vi "table_control.vi"() -> ()   [LabVIEW 2018]
uses:
  <vilib>/Utility/miscctls.llb/LVRowAndColumnUnsignedTypeDef.ctl
panel:
  in  "Stop":bool
  out "Loop Index":i32
  in  "Table Control":string[][](table)
  # "Adapted from\nhttps://www.youtube.com/watch?v=RbDLJ1aaG3E"
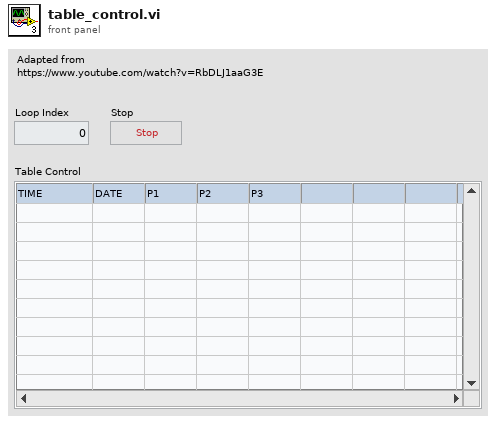
[diagram p1: front panel]
types:
  T1 = typedef "LVRowAndColumnUnsignedTypeDef.ctl" = cluster{"Row":u32, "Column":u32}
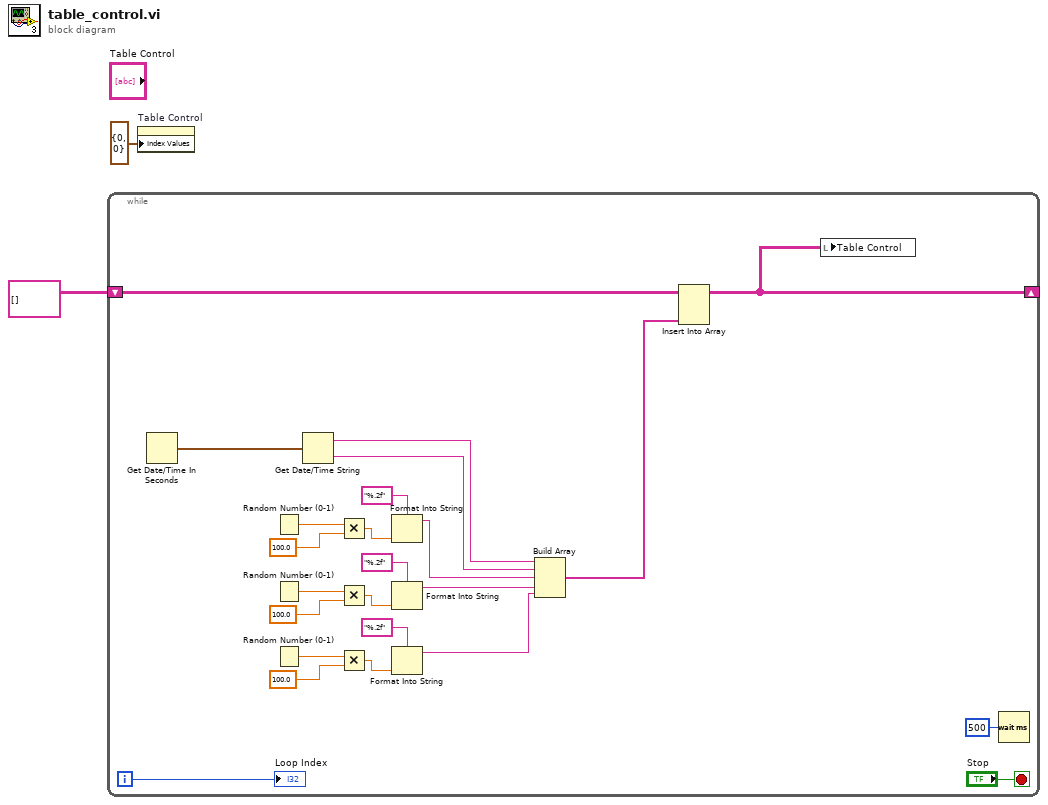
[diagram p0: block diagram]
diagram:
  n1 = while {
    shift-right: [w24] -> _
    shift-left: string[][] [] -> [w25]
    i -> [w26]
    stop <- "Stop" stop-if-true
    n2 = Get Date/Time In Seconds() -> (seconds since 1Jan1904=w6:timestamp)
    n3 = Random Number (0-1)() -> (number: 0 to 1=w23:dbl)
    n4 = Random Number (0-1)() -> (number: 0 to 1=w16:dbl)
    n5 = Random Number (0-1)() -> (number: 0 to 1=w15:dbl)
    n6 = Get Date/Time String(seconds (now)=w6) -> (date string=w7:string, time string=w8:string)  [unwired: 2 in]
    n7 = Multiply(x=w23, y=100.0) -> (x*y=w21:dbl)
    n8 = Multiply(x=w16, y=100.0) -> (x*y=w18:dbl)
    n9 = Multiply(x=w15, y=100.0) -> (x*y=w13:dbl)
    n10 = Format Into String(format string="%.2f", w21) -> (resulting string=w10:string)  [unwired: 2 in, 1 out]
    n11 = Format Into String(format string="%.2f", w18) -> (resulting string=w9:string)  [unwired: 2 in, 1 out]
    n12 = Format Into String(format string="%.2f", w13) -> (resulting string=w11:string)  [unwired: 2 in, 1 out]
    n13 = Build Array(w7, w8, w10, w9, w11) -> (w5:string[])
    n14 = Insert Into Array(array=w25, new element=w5) -> (w24:string[][])  [unwired: 2 in]
    n15 = local write "Table Control"(w24) -> ()
    n16 = Wait (ms)(milliseconds to wait=u32 500) -> ()  [unwired: 1 out]
    "Loop Index" <- w26
  }
  n17 = property on="Table Control" class="Tbl (strict)"("Index Values"=T1 {"Row"=0, "Column"=0}) -> ()  [unwired: 2 in, 2 out]
